vi "AdjustPIDParameters_subVI.vi"() -> ()   [LabVIEW 2015, in "JULABO DeviceDriver.lvlib"]
doc: "This example shows how to change control parameters in the unit"
uses:
  <instrlib>/JULABO DeviceDriver/JULABO DeviceDriver.lvlib
panel:
  out "error out":errorcluster caption="Fehler (Ausgang)"
  in  "Adjust":bool
  in  "Tv (0s)":u16 max=999
  in  "Tn (3s)":u16=3 min=3 max=9999
  in  "Xp (0.6K)":dbl=0.6 min=0.1 max=99.9
  out "Selftuning (out)":enum16{"OFF", "ONCE", "ALWAYS"}(ring)
  out "InternalTv (out)":u16
  out "InternalTn (out)":u16
  out "InternalXp (out)":dbl
  in  "VISA resource name":refnum<visa-resource-name>="COM3"
  in  "Reset / Default (T: Both)":bool=TRUE
  in  "ID Query? (T: Yes)":bool=TRUE
  in  "RS485-Address (128: RS232)":u32=128
  in  "Serial Configuration":T1={"Baud Rate"=4800, "Parity"=2, "Data Bits"=7, "Stop Bits"=10, "Flow Control"=2} {"Flow Control" items=["None", "XON/XOFF", "RTS/CTS", "XON/XOFF & RTS/CTS", "DTR/DSR", "XON/XOFF & DTR/DSR"]; "Stop Bits" items=["1.0"=10, "1.5"=15, "2.0"=20]; "Data Bits" items=["7"=7, "8"=8]; "Parity" items=["None", "Odd", "Even", "Mark", "Space"]; "Baud Rate" items=["300"=300, "600"=600, "1200"=1200, "2400"=2400, "4800"=4800, "9600"=9600, "19200"=19200]}
  # "1. Select the COM-Port and adjust the serial\nconfiguration for your instrument\n2. Adjust the Read cycle\n3. Start the VI by pressing the \"Start\" -Button\n( Arrow button on the top-left corner)\n4. To stop the execution press the \"Stop\" button"
  # "Adjust parameters"
  # "Read parameters"
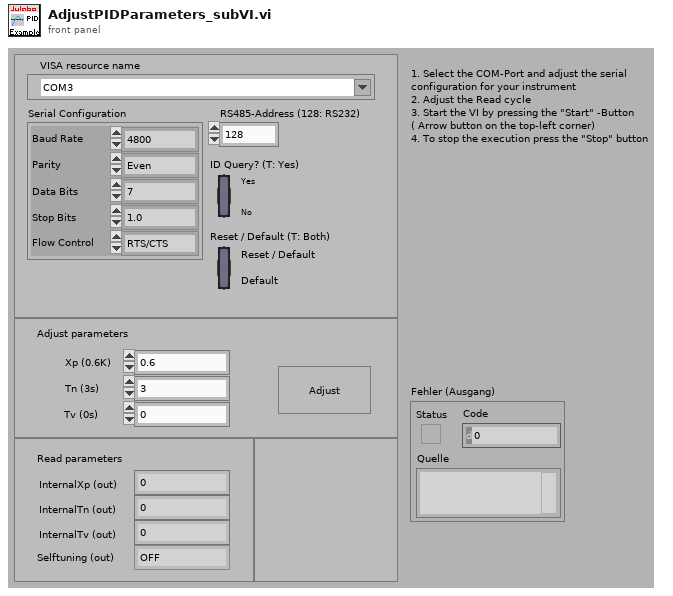
[diagram p1: front panel]
types:
  T1 = cluster{"Baud Rate":u32, "Parity":u16, "Data Bits":u16, "Stop Bits":u16, "Flow Control":u16}
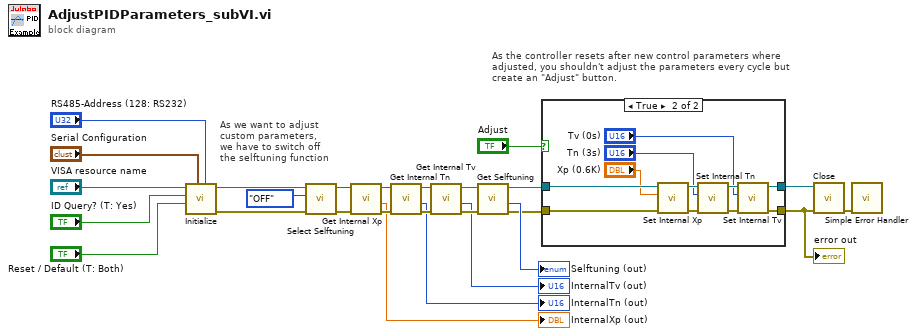
[diagram p0: block diagram]
diagram:
  # "As the controller resets after new control parameters where\nadjusted, you shouldn't adjust the parameters every cycle but\ncreate an \"Adjust\" button."
  # "As we want to adjust\ncustom parameters,\nwe have to switch off\nthe selftuning function"
  n1 = call <instrlib>:"Initialize.vi"("RS485-Address (128: RS232)"="RS485-Address (128: RS232)", "Serial Configuration"="Serial Configuration", "Reset / Default (T: Both)"="Reset / Default (T: Both)", "ID Query? (T: Yes)"="ID Query? (T: Yes)", "VISA resource name"="VISA resource name") -> ("error out"=w17:errorcluster, "VISA resource name out"=w18:refnum<visa-resource-name>)  [unwired: 5 in]
  n2 = call "Select Selftuning.vi"("error in (no error)"=w17, "Selftuning (0: OFF)"=enum16{"OFF", "ONCE", "ALWAYS"}."OFF", "VISA resource name"=w18) -> ("error out"=w1:errorcluster, "VISA resource name out"=w16:refnum<visa-resource-name>)  [unwired: 7 in]
  n3 = call <instrlib>:"Get Internal Xp.vi"("error in"=w1, "VISA resource name in"=w16) -> ("error out"=w13:errorcluster, "InternalXp (out)"=→"InternalXp (out)":dbl, "VISA resource name out"=w14:refnum<visa-resource-name>)  [unwired: 7 in]
  n4 = call <instrlib>:"Get Internal Tn.vi"("error in"=w13, "VISA resource name in"=w14) -> ("error out"=w11:errorcluster, "InternalTn (out)"=→"InternalTn (out)":u16, "VISA resource name out"=w12:refnum<visa-resource-name>)  [unwired: 7 in]
  n5 = call <instrlib>:"Get Internal Tv.vi"("error in"=w11, "VISA resource name in"=w12) -> ("error out"=w9:errorcluster, "InternalTv (out)"=→"InternalTv (out)":u16, "VISA resource name out"=w10:refnum<visa-resource-name>)  [unwired: 7 in]
  n6 = call "Get Selftuning.vi"("error in"=w9, "VISA resource name in"=w10) -> ("error out"=w3:errorcluster, "Selftuning (out)"=→"Selftuning (out)":enum16{"OFF", "ONCE", "ALWAYS"}, "VISA resource name out"=w4:refnum<visa-resource-name>)  [unwired: 7 in]
  n7 = case shown="True" "Adjust" {
    tunnel: w4 -> [w28 w35]
    tunnel: w3 -> [w27 w34]
    tunnel: [w28 w33] -> w26
    tunnel: [w27 w32] -> w25
    frame False {
    }
    frame True {
      n8 = call <instrlib>:"Set Internal Xp.vi"("error in (no error)"=w34, "Xp (0.6K)"="Xp (0.6K)", "VISA resource name"=w35) -> ("error out"=w37:errorcluster, "VISA resource name out"=w36:refnum<visa-resource-name>)  [unwired: 7 in]
      n9 = call <instrlib>:"Set Internal Tn.vi"("error in (no error)"=w37, "Tn (3s)"="Tn (3s)", "VISA resource name"=w36) -> ("error out"=w39:errorcluster, "VISA resource name out"=w38:refnum<visa-resource-name>)  [unwired: 7 in]
      n10 = call <instrlib>:"Set Internal Tv.vi"("error in (no error)"=w39, "Tv (0s)"="Tv (0s)", "VISA resource name"=w38) -> ("error out"=w32:errorcluster, "VISA resource name out"=w33:refnum<visa-resource-name>)  [unwired: 7 in]
    }
  }
  "error out" <- w25
  n11 = call <instrlib>:"Close.vi"("error in (no error)"=w25, "VISA resource name"=w26) -> ("error out"=w22:errorcluster)  [unwired: 9 in]
  n12 = call <vilib>:"Simple Error Handler.vi"("error in (no error)"=w22) -> ()  [unwired: 4 in, 5 out]
